vi "Actor Core.vi"(8 "error in":errorcluster, 11 "Assembly Run in":refnum<class "Assembly Run.lvclass">) -> (0 "error out":errorcluster, 3 "Actor out":refnum<class "Actor.lvclass">)   [LabVIEW 2021, in "Assembly Run.lvclass"]
doc: "(<B>Filename</B>: Actor Framework.lvlib:Actor.lvclass:Actor Core.vi)\n\nReceives messages to the actor, reacts to them, and initiates any error handling that may shut the actor down.\n\nDescendant classes may override this VI to append parallel tasks for the actor to complete while it handles messages. Overrides use the Call Parent Class Method node."
uses:
  Assembly Run.lvclass
  C:/Program Files (x86)/National Instruments/LabVIEW 2021/vi.lib/ActorFramework/Actor/Actor.lvclass
  <vilib>/ActorFramework/Actor/Actor.lvclass
  Routine/Routine Enum.ctl
  Workspace/Fixture Enum.ctl
  <vilib>/ActorFramework/Message Enqueuer/Message Enqueuer.lvclass
  Workspace/Fixture.lvclass
  Routine/Routine.lvclass
panel:
  in  "Stop Button":bool
  in  "Fixtures":T1[](array[typedef])
  in  "Routines":T2[](array[typedef])
  in  "run":bool
  in  "find centers":bool
  in  "add":bool
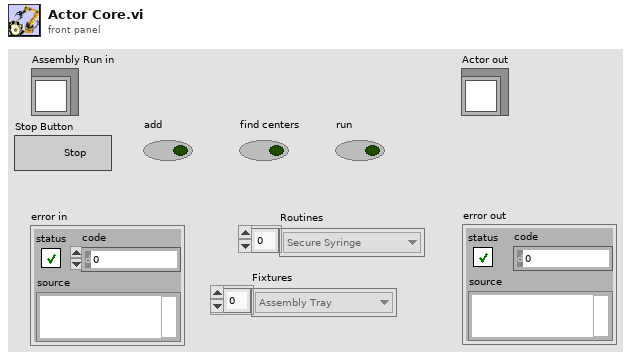
[diagram p1: front panel]
types:
  T1 = typedef "Fixture.lvclass/Fixture Enum.ctl" = enum16{"Assembly Tray", "Syringe Space", "Component", "Pick Up Tool", "Current Position"}
  T2 = typedef "Routine.lvclass/Routine Enum.ctl" = enum16{"Primary Pick Up", "Secondary Pick Up", "Put Down All", "Secure Syringe", "Release Syringe", "Dispense on Plate", "Dispense on Sensor", "Pick Up All", "Put Down Secondary", "Dispense on Kapton", "Full Assembly"}
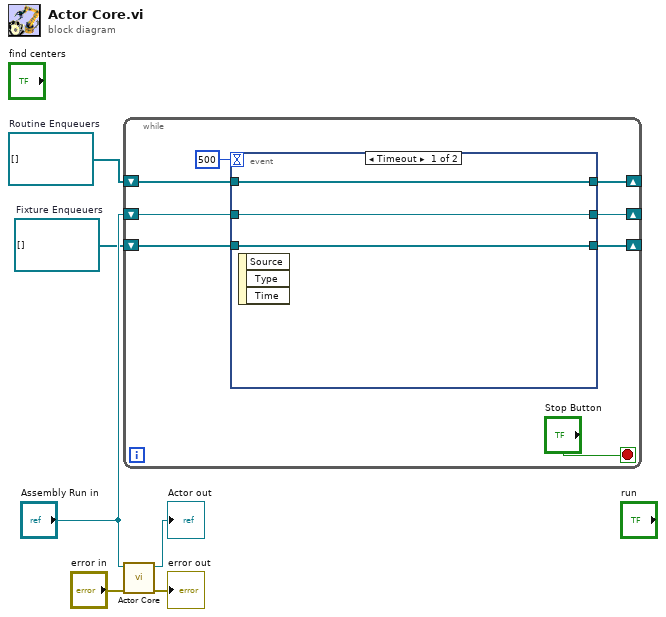
[diagram p0: block diagram]
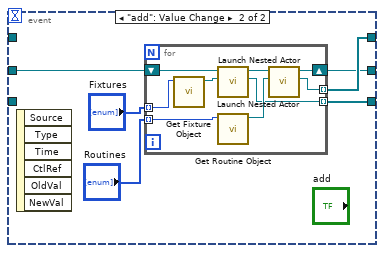
[diagram p2: hidden frame]
diagram:
  w1 = refnum<class "Message Enqueuer.lvclass">[] []  # Routine Enqueuers
  w2 = refnum<class "Message Enqueuer.lvclass">[] []  # Fixture Enqueuers
  n1 = while {
    shift-right: [w8] -> _
    shift-left: "Assembly Run in" -> [w14]
    shift-right: [w12] -> _
    shift-left: w2 -> [w11]
    shift-right: [w13] -> _
    shift-left: w1 -> [w10]
    stop <- "Stop Button" stop-if-true
    n2 = event shown="[0] Timeout" {
      selector: _ -> [_ _]
      dyn-events: _ -> [_ _]
      timeout: 500 -> [_ _]
      tunnel: w14 -> [w15 w21]
      tunnel: [w16 w20] -> w13
      tunnel: [w17 w19] -> w12
      tunnel: w11 -> [w17 _]
      tunnel: w10 -> [w16 _]
      tunnel: [w15 w18] -> w8
      event Timeout {
        n3 = event-data() -> ()  [unwired: 1 in, 3 out]
      }
      event "add": Value Change {
        n4 = event-data() -> ()  [unwired: 1 in, 6 out]
        n5 = for {
          tunnel: "Routines" -> [w32] mode=indexing
          tunnel: "Fixtures" -> [w31] mode=indexing
          shift-right: [w27] -> w18
          shift-left: w21 -> [w29]
          tunnel: [w25] -> w19 mode=indexing
          tunnel: [w24] -> w20 mode=indexing
          n6 = call "Get Fixture Object.vi"("Fixture"=w31) -> ("Workspace.lvclass"=w30:refnum<class "Fixture.lvclass">)  [unwired: 8 in, 2 out]
          n7 = call <vilib>:"Launch Nested Actor.vi"("Nested Actor"=w30, "Caller Actor in"=w29) -> ("Nested Actor's Enqueuer"=w25:refnum<class "Message Enqueuer.lvclass">, "Caller Actor out"=w28:refnum<class "Assembly Run.lvclass">)  [unwired: 7 in, 1 out]
          n8 = call "Get Routine Object.vi"("Routine"=w32) -> ("Routine out"=w26:refnum<class "Routine.lvclass">)  [unwired: 9 in, 1 out]
          n9 = call <vilib>:"Launch Nested Actor.vi"("Nested Actor"=w26, "Caller Actor in"=w28) -> ("Nested Actor's Enqueuer"=w24:refnum<class "Message Enqueuer.lvclass">, "Caller Actor out"=w27:refnum<class "Assembly Run.lvclass">)  [unwired: 7 in, 1 out]
        }
      }
    }
  }
  n10 = call-parent "Actor Core.vi"("error in"="error in", "Actor in"="Assembly Run in") -> ("error out"=→"error out":errorcluster, "Actor out"=→"Actor out":refnum<class "Actor.lvclass">)  [unwired: 8 in]
